vi "Network Steam Create.vi"(8 "error in (no error)":errorcluster, 11 "Model in":refnum<class "Model.lvclass">) -> (0 "error out":errorcluster, 3 "Model out":refnum<class "Model.lvclass">)   [LabVIEW 2021, in "Model.lvlib" / "Model.lvclass"]
uses:
  Model.lvclass
  <userlib>/John_Lib/Network_Streams_Connection/PublicSettings.ctl
  Model.lvclass/Model.ctl
  <userlib>/John_Lib/Network_Streams_Connection/NetworkConnection.lvclass
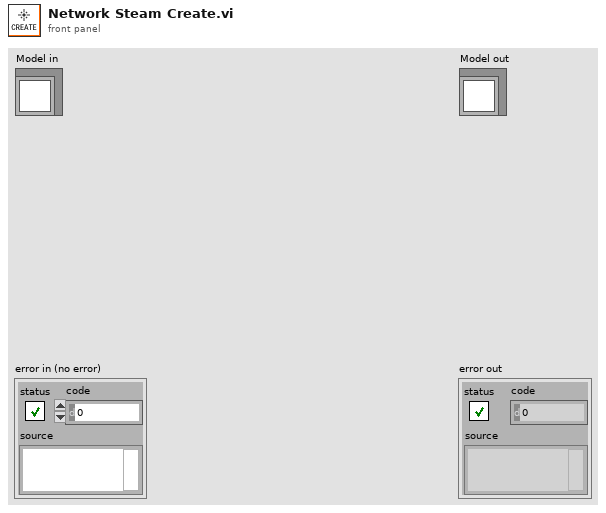
[diagram p1: front panel]
types:
  T1 = typedef "JKI_Network_Streams.lvlib/NetworkConnection.lvclass/PublicSettings.ctl" = cluster{"My Name":string, "Remote IP Address":string, "Remote Name":string}
  T2 = typedef "Model.lvlib/Model.lvclass/DVR.ctl" = cluster{"JKI_Network_Streams":refnum<class "NetworkConnection.lvclass">}
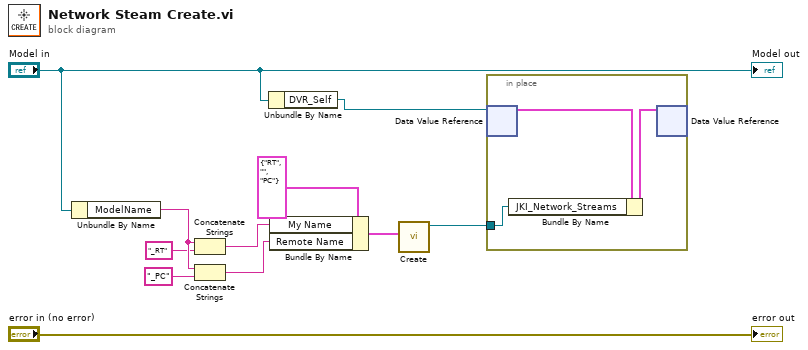
[diagram p0: block diagram]
diagram:
  n1 = Unbundle By Name("Model in") -> ("ModelName"=w10:string)
  n2 = Concatenate Strings(w10, "_RT" ("string")) -> (w7:string)
  n3 = Concatenate Strings(w10, "_PC" ("string")) -> (w9:string)
  n4 = Unbundle By Name("Model in") -> ("DVR_Self"=w2:refnum<data-value>)
  n5 = Bundle By Name(cluster=T1 {"My Name"="RT", "Remote IP Address"="", "Remote Name"="PC"} ("Settings"), "My Name"=w7, "Remote Name"=w9) -> (w5:T1)
  n6 = call <userlib>:"Create.vi"("Settings"=w5) -> ("NetworkConnection out"=w1:refnum<class "NetworkConnection.lvclass">)  [unwired: 9 in, 1 out]
  n7 = in-place {
    in-place-border: w1 -> [w12]
    n8 = in-place-dvr #1(w2) -> (w14:T2)  [unwired: 1 out]
    n9 = Bundle By Name(cluster=w14, "JKI_Network_Streams"=w12) -> (w13:T2)
    n10 = in-place-dvr #1(w13) -> ()  [unwired: 2 out]
  }
  "error out" <- "error in (no error)"
  "Model out" <- "Model in"
